vi "SLSC Convert EDS Command to Tree Control Item.vi"(11 "command":T1) -> (2 "Glyph":i32, 3 "Child Text":string[](array[string]))   [LabVIEW 2020, in "SLSC Tree Control.lvlib"]
doc: "Convert the EDS property datatype to a Tree Control Child Text."
uses:
  SLSC Tree Control.lvlib
  SLSC EDS API/JSON parsing/command.ctl
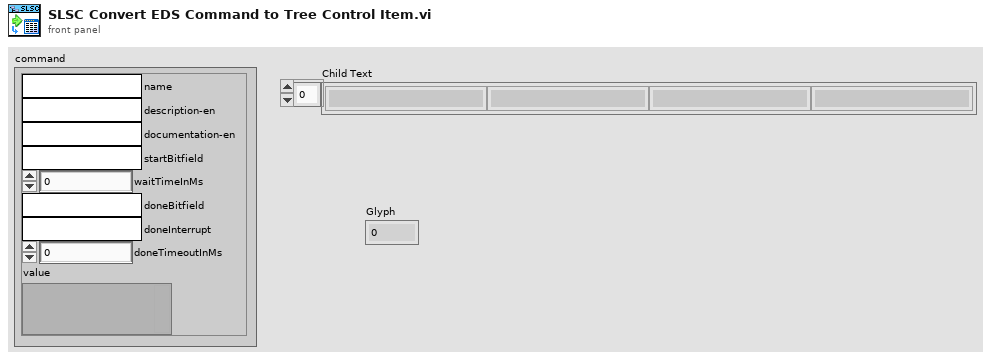
[diagram p1: front panel]
types:
  T1 = typedef "command.ctl" = cluster{"name":string, "description-en":string, "documentation-en":string, "startBitfield":string, "waitTimeInMs":i32, "doneBitfield":string, "doneInterrupt":string, "doneTimeoutInMs":i32, "value":variant}
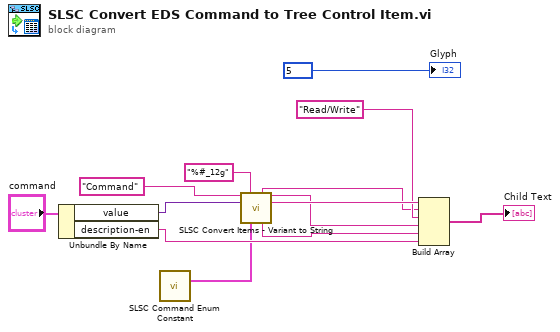
[diagram p0: block diagram]
diagram:
  n1 = Unbundle By Name("command") -> ("value"=w11:variant, "description-en"=w2:string)
  n2 = call "SLSC Command Enum Constant.vi"() -> ("String Enums"=w1:cluster{"name":string, "string enums":string}[])  [unwired: 11 in, 4 out]
  n3 = call "SLSC Convert Items - Variant to String.vi"("Datatype"="Command" ("dataType"), "format string"="%#_12g", "value"=w11, "Enum string"=w1) -> ("string data reset value"=w3:string, "Output data type"=w7:string, "string data value"=w8:string, "enum_range"=w9:string)  [unwired: 5 in, 3 out]
  n4 = Build Array(w8, w3, "Read/Write" ("element"), w7, w9, w2) -> (→"Child Text":string[])
  "Glyph" <- 5
